vi "Build Tx-Generic Cluster.vi"(8 "error in":errorcluster, 9 "port properties":T1, 10 "board properties":T2 {"portConfig" items=["FDX_SINGLE", "FDX_REDUNDANT"]; "portSpeed" items=["FDX_100MBIT", "FDX_10MBIT", "FDX_AUTO_100MBIT", "FDX_AUTO_10MBIT", "FDX_AUTO_ERROR", "FDX_1000MBIT"]}, 11 "section ref in":T7=18446744073709551615 format="%.0x") -> (0 "error out":errorcluster, 2 "Tx cluster out":T3 {"channel settings"."Frame Array"."Data" format="%.0x"; "channel settings"."Frame Array"."HeaderInfo"."NetSelect" items=["FDX_TX_FRAME_DLY_A"=0, "FDX_TX_FRAME_DLY_B"=1, "FDX_TX_FRAME_BOTH "=3, "FDX_TX_FRAME_ONLY_A"=4, "FDX_TX_FRAME_ONLY_B "=5]; "channel settings"."Frame Array"."HeaderInfo"."FrameStartMode" items=["FDX_TX_FRAME_START_IFG", "FDX_TX_FRAME_START_PGWT", "FDX_TX_FRAME_START_TRG"]; "channel settings"."Frame Array"."HeaderInfo"."PhysErrorInjection" items=["FDX_TX_FRAME_ERR_OFF"=0, "FDX_TX_FRAME_ERR_CRC"=1, "FDX_TX_FRAME_ERR_ALI"=2, "FDX_TX_FRAME_ERR_PRE"=4, "FDX_TX_FRAME_ERR_PHY"=8]; "channel settings"."Frame Array"."HeaderInfo"."SequenceNumberInit" items=["FDX_TX_FRAME_SEQ_INIT_AUTO"=65535]; "channel settings"."Frame Array"."HeaderInfo"."SequenceNumberOffset" items=["FDX_TX_FRAME_SEQ_OFFS_AUTO "=65535]; "channel settings"."Frame Array"."HeaderInfo"."PayloadGenerationMode" items=["FDX_TX_FRAME_PGM_USER"=0, "FDX_TX_FRAME_PGM_IP_PART"=1, "FDX_TX_FRAME_PGM_IP_FULL"=2, "FDX_TX_FRAME_PGM_IP_PART_TT"=10, "FDX_TX_FRAME_PGM_IP_FULL_TT"=20]; "channel settings"."Frame Array"."HeaderInfo"."PayloadBufferMode" items=["FDX_TX_FRAME_PBM_STD", "FDX_TX_FRAME_PBM_MAC", "FDX_TX_FRAME_PBM_UDP"]}, 3 "section ref out":T7 format="%.0x")   [LabVIEW 2020, in "AIM ARINC 664 Scripting.lvlib"]
uses:
  AIM ARINC 664 Scripting.lvlib
  <vilib>/NI VeriStand/Custom Device API/Custom Device Item Ref.ctl
  Engine/Implementation/Tx Execution Unit/hardware_channels_tx.ctl
  Engine/Implementation/Tx Execution Unit/channel_settings_tx.ctl
  Shared/RawFrame.ctl
  <instrlib>/AIM GmbH/_AIM 664/_controls/queue_header_generic.ctl
  Shared/board_setup.ctl
  Shared/port_setup.ctl
  Shared/session_tx_generic.ctl
  <instrlib>/AIM GmbH/_AIM 664/AIM664LV.lvlib
  Engine/Implementation/Tx Execution Unit/Tx Generic Execution Unit.lvclass
  <vilib>/Utility/SystemLogging/NI_SystemLogging.lvlib
  Import/AIM ARINC 664 Import.lvlib
  <vilib>/NI VeriStand/Custom Device API/Custom Device API.lvlib
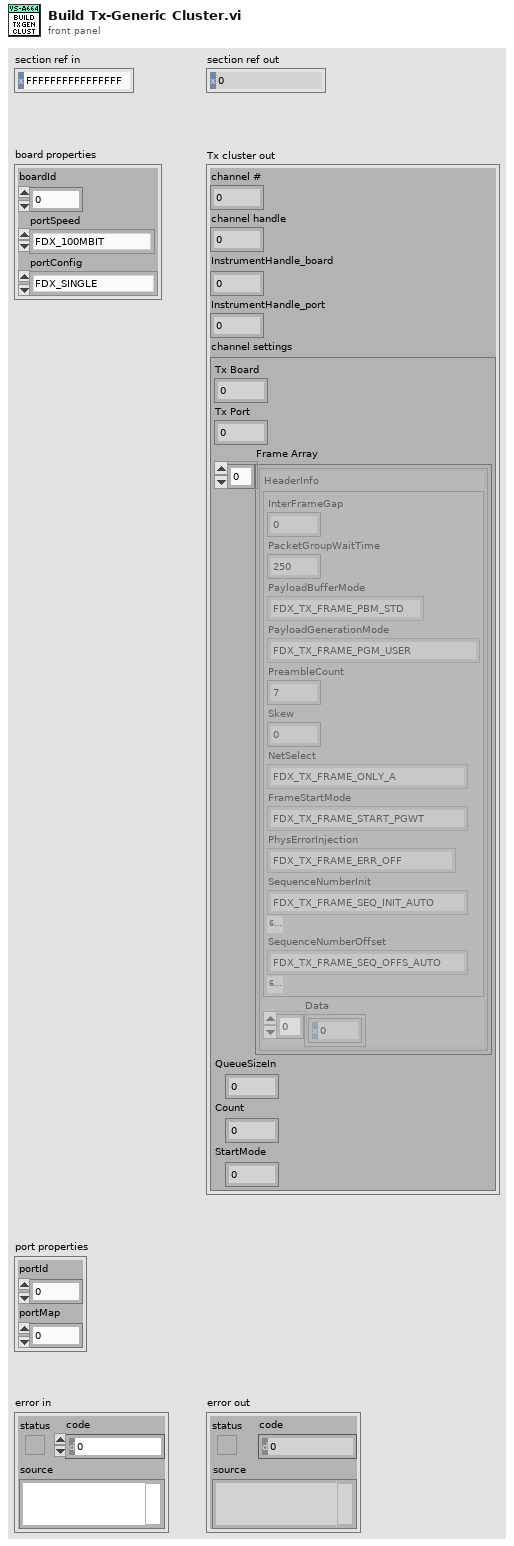
[diagram p1: front panel]
types:
  T1 = typedef "AIM ARINC 664 Import.lvlib/port_setup.ctl" = cluster{"portId":u32, "portMap":u32}
  T2 = typedef "AIM ARINC 664 Import.lvlib/board_setup.ctl" = cluster{"boardId":u32, "portSpeed":u32, "portConfig":u32}
  T3 = typedef "AIM ARINC 664 Engine.lvlib/Implementation.lvlib/Tx Generic Execution Unit.lvclass/hardware_channels_tx.ctl" = cluster{"channel #":u16, "channel handle":u64, "InstrumentHandle_board":u32, "InstrumentHandle_port":u32, "channel settings":T4}
  T4 = typedef "AIM ARINC 664 Engine.lvlib/Implementation.lvlib/Tx Generic Execution Unit.lvclass/channel_settings_tx.ctl" = cluster{"Tx Board":u32, "Tx Port":u32, "Frame Array":T5[], "QueueSizeIn":u32, "Count":u32, "StartMode":u32}
  T5 = typedef "RawFrame.ctl" = cluster{"HeaderInfo":T6, "Data":u8[]}
  T6 = typedef "AIM664LV.lvlib/queue_header_generic.ctl" = cluster{"InterFrameGap":u32, "PacketGroupWaitTime":u32, "PayloadBufferMode":u8, "PayloadGenerationMode":u8, "PreambleCount":u8, "Skew":u32, "NetSelect":u8, "FrameStartMode":u8, "PhysErrorInjection":u32, "SequenceNumberInit":u16, "SequenceNumberOffset":u16}
  T7 = typedef "Custom Device API.lvlib/Custom Device Item Ref.ctl" = u64
  T8 = typedef "AIM ARINC 664 Import.lvlib/session_tx_generic.ctl" = cluster{"QueueSizeIn":u32, "Count":i32, "StartMode":i32}
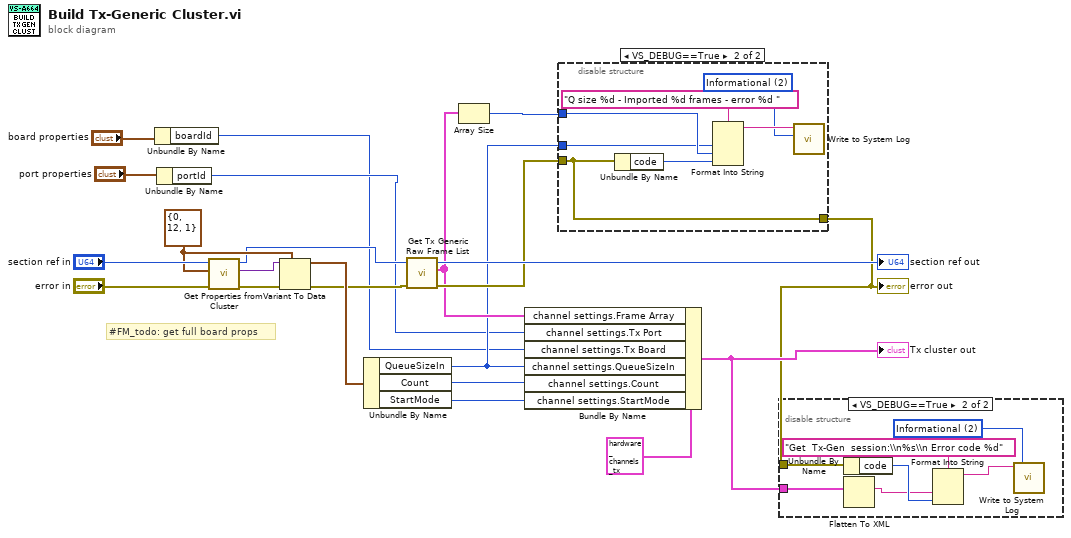
[diagram p0: block diagram]
diagram:
  w14 = T8 {"QueueSizeIn"=0, "Count"=12, "StartMode"=1} ("session_tx_generic")
  # "#FM_todo: get full board props"
  n1 = Unbundle By Name("board properties") -> ("boardId"=w3:u32)
  n2 = Unbundle By Name("port properties") -> ("portId"=w5:u32)
  n3 = call "Get Properties from Cluster.vi"("error in"="error in", "Variant Cluster"=w14, "custom device ref in"="section ref in") -> ("error out"=w13:errorcluster, "data"=w15:variant, "custom device ref out"=w10:T7)  [unwired: 5 in, 1 out]
  n4 = Variant To Data(error in=w13, type=w14, Variant=w15) -> (data=w12:T8, error out=w11:errorcluster)
  n5 = Unbundle By Name(w12) -> ("QueueSizeIn"=w7:u32, "Count"=w8:i32, "StartMode"=w9:i32)
  n6 = call "Get Tx Generic Raw Frame List.vi"("error in"=w11, "custom device ref in"=w10) -> ("error out"=w18:errorcluster, "Raw Frame List"=w17:T5[], "custom device ref out"=→"section ref out":T7)  [unwired: 6 in, 1 out]
  n7 = Array Size(array=w17) -> (size(s)=w16:i32)
  n8 = Bundle By Name(cluster=T3 {"channel #"=0, "channel handle"=0, "InstrumentHandle_board"=0, "InstrumentHandle_port"=0, "channel settings"={"Tx Board"=0, "Tx Port"=0, "Frame Array"=[{"HeaderInfo"={"InterFrameGap"=0, "PacketGroupWaitTime"=250, "PayloadBufferMode"=0, "PayloadGenerationMode"=0, "PreambleCount"=7, "Skew"=0, "NetSelect"=4, "FrameStartMode"=1, "PhysErrorInjection"=0, "SequenceNumberInit"=65535, "SequenceNumberOffset"=65535}, "Data"=[]}, {"HeaderInfo"={"InterFrameGap"=0, "PacketGroupWaitTime"=250, "PayloadBufferMode"=0, "PayloadGenerationMode"=0, "PreambleCount"=7, "Skew"=0, "NetSelect"=4, "FrameStartMode"=1, "PhysErrorInjection"=0, "SequenceNumberInit"=65535, "SequenceNumberOffset"=65535}, "Data"=[]}], "QueueSizeIn"=0, "Count"=0, "StartMode"=0}} ("TX Parameters"), "channel settings.Frame Array"=w17, "channel settings.Tx Port"=w5, "channel settings.Tx Board"=w3, "channel settings.QueueSizeIn"=w7, "channel settings.Count"=w8, "channel settings.StartMode"=w9) -> (w2:T3)
  "Tx cluster out" <- w2
  n9 = disable-structure shown="VS_DEBUG==True" {
    disable-tunnel: w18 -> [_ w24]
    disable-tunnel: w16 -> [_ w25]
    disable-tunnel: [_ w24] -> w1
    disable-tunnel: w7 -> [_ w23]
    frame condition #0 {
    }
    frame condition #1 (active) {
      w27 = 2 items=["Error", "Warning", "Informational"] ("severity")
      n10 = Unbundle By Name(w24) -> ("code"=w26:i32)
      n11 = Format Into String(format string="Q size %d - Imported %d frames - error %d ", w23, w25, w26) -> (resulting string=w28:string)  [unwired: 2 in, 1 out]
      n12 = call <vilib>:"Write to System Log.vi"("severity"=w27, "message"=w28) -> ()  [unwired: 9 in, 1 out]
    }
  }
  "error out" <- w1
  n13 = disable-structure shown="VS_DEBUG==True" {
    disable-tunnel: w1 -> [_ w32]
    disable-tunnel: w2 -> [_ w31]
    frame condition #0 {
    }
    frame condition #1 (active) {
      w34 = 2 items=["Error", "Warning", "Informational"] ("severity")
      n14 = Unbundle By Name(w32) -> ("code"=w33:i32)
      n15 = Flatten To XML(6:w31) -> (2:w30:string)
      n16 = Format Into String(format string="Get  Tx-Gen  session:\\n%s\\n Error code %d", w30, w33) -> (resulting string=w35:string)  [unwired: 2 in, 1 out]
      n17 = call <vilib>:"Write to System Log.vi"("severity"=w34, "message"=w35) -> ()  [unwired: 9 in, 1 out]
    }
  }
